vi "WriteConfigIniCluster.vi"(0 "更随产品型号变更？":bool, 1 "ConfigFlieName":string="信号循环发送接收参数.ini", 2 "ConfigIn":variant, 3 "ProductName":string="产品名称XXX", 5 "error in (no error)":errorcluster caption="错误输入（无错误）") -> (19 "error out":errorcluster caption="错误输出")   [LabVIEW 2020]
doc: "如果参数文件不跟产品型号走，就不需要填ProductName"
uses:
  <vilib>/Utility/config.llb/NI_LVConfig.lvlib
  DAQ_Base.lvclass
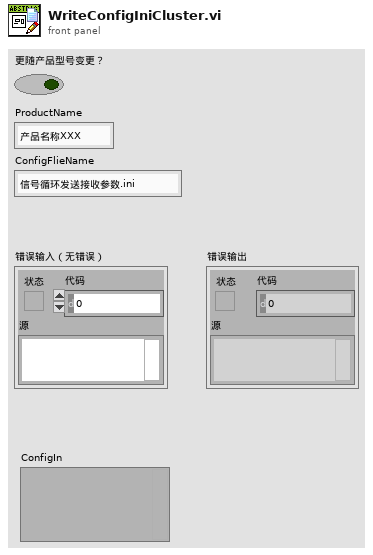
[diagram p1: front panel]
types:
  T1 = typedef "NI_LVConfig.lvlib/Config Data RefNum.ctl" = refnum<k1>
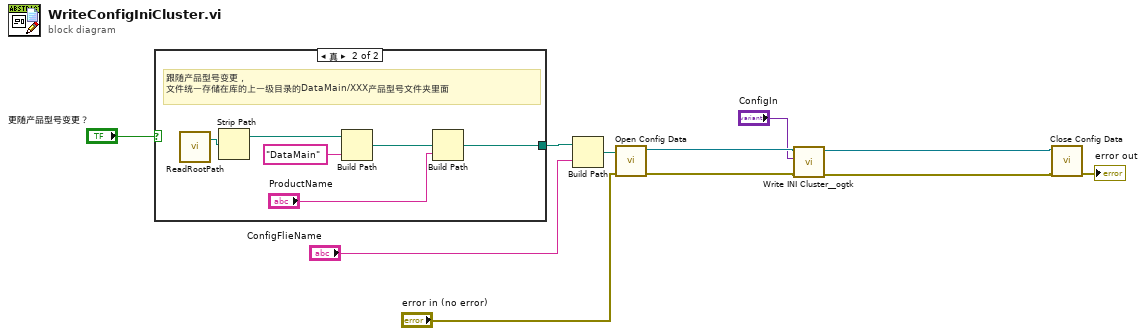
[diagram p0: block diagram]
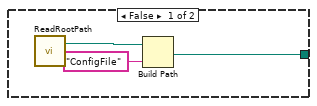
[diagram p2: hidden frame]
diagram:
  n1 = case shown="真" "更随产品型号变更？" {
    tunnel: [w12 w16] -> w10
    frame False {
      n2 = call "ReadRootPath.vi"() -> ("Root path"=w13:path)  [unwired: 19 in]
      n3 = Build Path(base path=w13, name or relative path="ConfigFile" ("ConfigFlieFolderName")) -> (appended path=w12:path)
    }
    frame True {
      # "跟随产品型号变更，\n文件统一存储在库的上一级目录的DataMain/XXX产品型号文件夹里面"
      n4 = call "ReadRootPath.vi"() -> ("Root path"=w18:path)  [unwired: 19 in]
      n5 = Strip Path(path=w18) -> (stripped path=w19:path)  [unwired: 1 out]
      n6 = Build Path(base path=w19, name or relative path="DataMain" ("ConfigFlieFolderName")) -> (appended path=w17:path)
      n7 = Build Path(base path=w17, name or relative path="ProductName") -> (appended path=w16:path)
    }
  }
  n8 = Build Path(base path=w10, name or relative path="ConfigFlieName") -> (appended path=w9:path)
  n9 = call <vilib>:"Open Config Data.vi"("error in (no error)"="error in (no error)", "configuration file path"=w9) -> ("error out"=w4:errorcluster, "refnum"=w5:T1)  [unwired: 7 in, 1 out]
  n10 = call <userlib>:"Write INI Cluster__ogtk.vi"("error in (no error)"=w4, "INI Fomatted Cluster"="ConfigIn", "refnum"=w5) -> ("error out"=w3:errorcluster, "dup refnum"=w2:T1)  [unwired: 7 in]
  n11 = call <vilib>:"Close Config Data.vi"("error in (no error)"=w3, "refnum"=w2) -> ("error out"=→"error out":errorcluster)  [unwired: 8 in, 1 out]
